vi "Generate IPs.vi"(8 "error in (no error)":errorcluster, 10 "Local Ip":string) -> (0 "error out":errorcluster, 2 "Search IP addresses":string[](array[string]))   [LabVIEW 2020, in "Controller.lvlib"]
uses:
  Controller.lvlib
panel:
  out "array":string[](array[string])
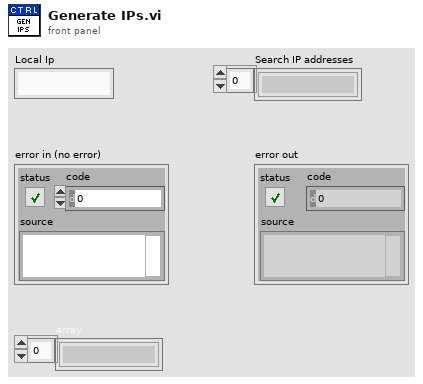
[diagram p1: front panel]
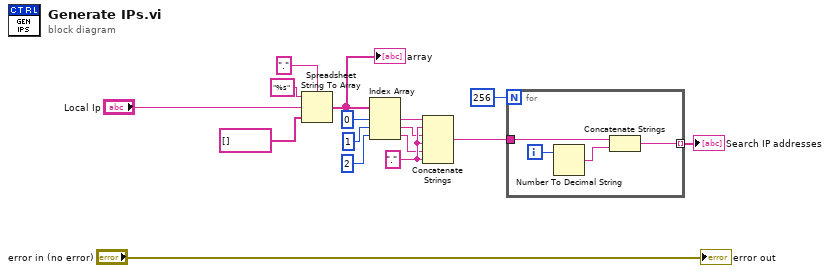
[diagram p0: block diagram]
diagram:
  w10 = "." ("delimiter (Tab)")
  n1 = Spreadsheet String To Array(delimiter (Tab)=".", format string="%s" ("spreadsheet string"), spreadsheet string="Local Ip", array type (2D Dbl)=string[] []) -> (array=w14:string[])
  "array" <- w14
  n2 = Index Array(array=w14, index #1=0 ("index"), index #2=1 ("index"), index #3=2 ("index")) -> (element #1=w9:string, element #2=w8:string, element #3=w7:string)
  n3 = Concatenate Strings(w9, w10, w8, w10, w7, w10) -> (w5:string)
  n4 = for {
    N: 256 -> [_]
    tunnel: w5 -> [w19]
    tunnel: [w20] -> w2 mode=indexing
    i -> [w17]
    n5 = Number To Decimal String(number=w17) -> (decimal integer string=w18:string)  [unwired: 1 in]
    n6 = Concatenate Strings(w19, w18) -> (w20:string)
  }
  "Search IP addresses" <- w2
  "error out" <- "error in (no error)"
